vi "determinePubDataSVs.vi"(8 "error in (no error)":errorcluster, 11 "MiddlewareSVThisComponent in":refnum<class "MiddlewareSVThisComponent.lvclass">) -> (0 "error out":errorcluster, 2 "svNames":string[](array[string]), 3 "MiddlewareSVThisComponent out":refnum<class "MiddlewareSVThisComponent.lvclass">)   [LabVIEW 2015, in "MiddlewareSVThisComponent.lvclass"]
uses:
  MiddlewareSVThisComponent.lvclass
  Typedefs/PubDataSV.ctl
  MiddlewareSVThisComponent.lvclass/MiddlewareSVThisComponent.ctl
  <vilib>/Utility/Data Type/NI_Data Type.lvlib
  Typedefs/EXATypedefs.lvlib
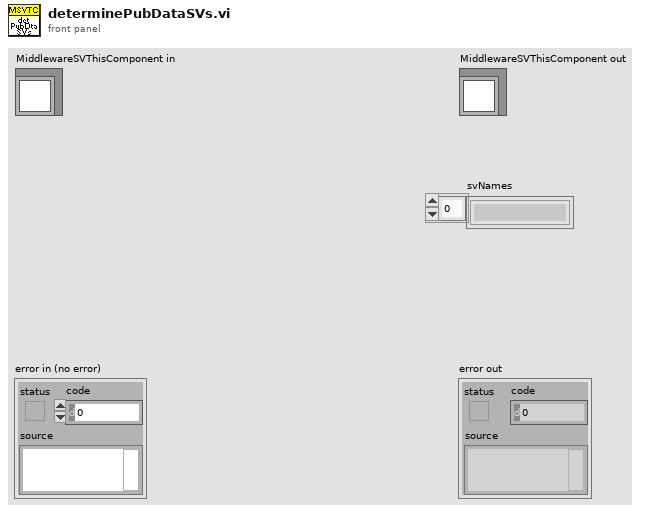
[diagram p1: front panel]
types:
  T1 = typedef "EXATypedefs.lvlib/PubDataSV.ctl" = enum16{"DetailedState", "ErrorCode", "Heartbeat", "LoopTime_ms", "LoopTimeOutOfRange", "RejectedCommand", "SummaryState", "Timestamp"}
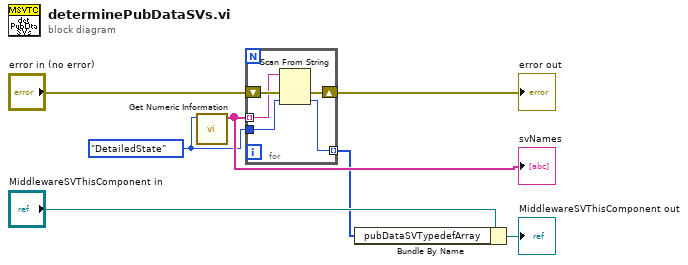
[diagram p0: block diagram]
diagram:
  w2 = PubDataSV."DetailedState" ("PubDataSV")
  n1 = call <vilib>:"Get Numeric Information.vi"("Variant"=w2) -> ("Enum Names"=w5:string[])  [unwired: 7 in, 3 out]
  "svNames" <- w5
  n2 = for {
    tunnel: [w11] -> w1 mode=indexing
    shift-right: [w9] -> w3
    shift-left: "error in (no error)" -> [w10]
    tunnel: w5 -> [w8] mode=indexing
    tunnel: w2 -> [w12]
    n3 = Scan From String(input string=w8, error in=w10, default 1=w12) -> (error out=w9:errorcluster, output 1=w11:T1)  [unwired: 2 in, 2 out]
  }
  "error out" <- w3
  n4 = Bundle By Name(cluster="MiddlewareSVThisComponent in", "pubDataSVTypedefArray"=w1) -> (→"MiddlewareSVThisComponent out":refnum<class "MiddlewareSVThisComponent.lvclass">)
